vi "Shutdown.vi"(7 "Error":errorcluster, 10 "FPGA VI Reference":refnum<k20>) -> (0 "Error Display":errorcluster)   [LabVIEW 2016]
uses:
  <vilib>/FPGAPlugInAG/myRIO-1900/niLvFpga_Close_myRIO-1900.vi
  <vilib>/rvi/interface/nirviCloseFPGA/nirviCloseFPGA.xnode
  <vilib>/NI_Real-Time Target Support.lvlib
  FPGA Bitfiles/Buggycompetition_FPGATarget2_AeroBuggyFPGA_9DbUQD1BP7s.lvbitx
  FPGA/FPGA.vi
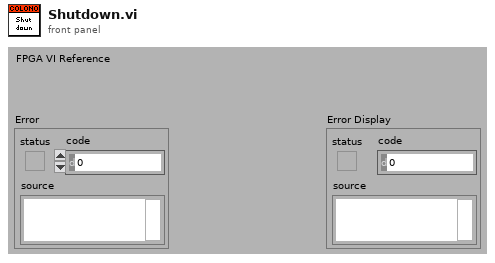
[diagram p1: front panel]
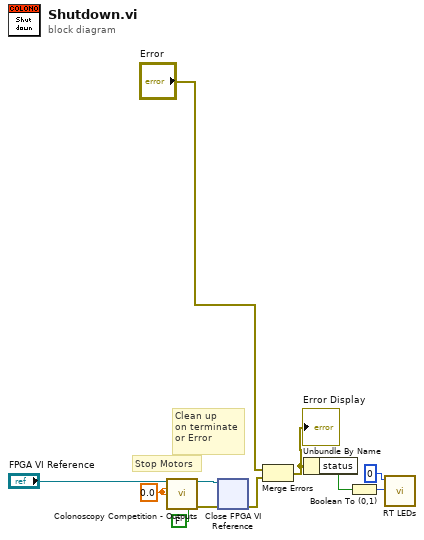
[diagram p0: block diagram]
diagram:
  w4 = 0.0 ("Motor 0 Control %")
  # "Clean up\non terminate\nor Error"
  # "Stop Motors"
  n1 = call "Colonoscopy Competition - Outputs.vi"("FPGA VI Reference"="FPGA VI Reference", "Motor 1 command"=w4, "Motor 2 command"=w4, "Enable motors?"=FALSE) -> ("FPGA VI Reference out"=w5:refnum<k20>, "Error Out"=w6:errorcluster)  [unwired: 10 in]
  n2 = xnode "Close FPGA VI Reference"("FPGA VI Reference In"=w5, "error in"=w6) -> ("error out"=w9:errorcluster)
  n3 = Merge Errors("Error", w9) -> (w11:errorcluster)
  "Error Display" <- w11
  n4 = Unbundle By Name(w11) -> ("status"=w10:bool)
  n5 = Boolean To (0,1)(Boolean=w10) -> (0, 1=w3:i16)
  n6 = call <vilib>:"RT LEDs.vi"("State"=w3, "LED Num"=0) -> ()  [unwired: 4 in, 2 out]
